vi "jl-script abs path.vi"(8 "error in (no error)":errorcluster, 10 "Base path (not a path)":path=path "", 11 "Julia user functions script":path) -> (0 "error out":errorcluster, 3 "script abs path":path)   [LabVIEW 2018, in "LV-0mq-Julia_roundtrip-lib.lvlib"]
doc: "If abs path is connected, this VI only checks if this file exists and puts the path through.\nFor a relative path, the abs path is constructed using the base path. \nIf base path not connected, the containing folder is assumed to be the \"jl-scripts\" folder in this LabVIEW library."
uses:
  LV-0mq-Julia_roundtrip-lib.lvlib
  <vilib>/Utility/error.llb/Error Cluster From Error Code.vi
  <vilib>/ErrorRing/Error Ring.xnode
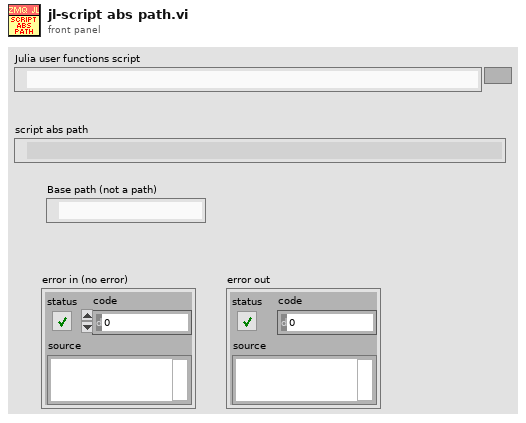
[diagram p1: front panel]
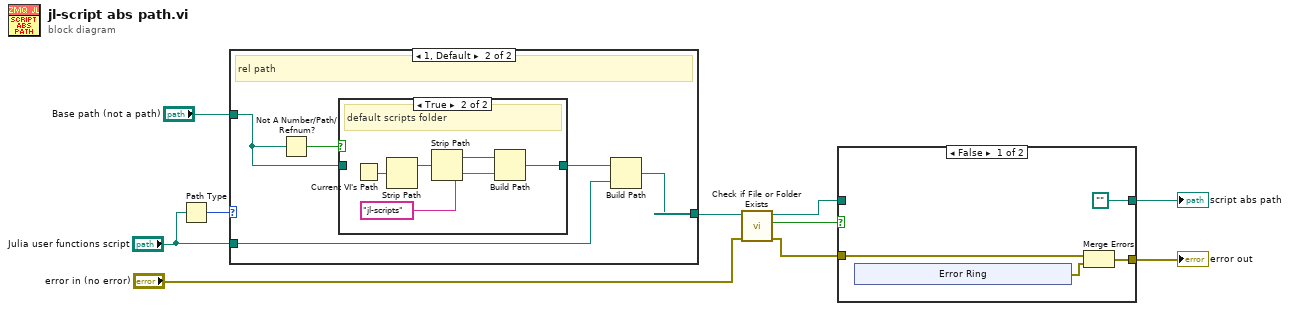
[diagram p0: block diagram]
diagram:
  n1 = Path Type(1:"Julia user functions script") -> (0:w3:i16)
  n2 = case shown="1, Default" w3 {
    tunnel: [w11 w16] -> w8
    tunnel: "Julia user functions script" -> [w11 w15]
    tunnel: "Base path (not a path)" -> [_ w12]
    frame 0 {
      # "abs path"
    }
    frame 1, Default {
      # "rel path"
      n3 = Not A Number/Path/Refnum?(number/path/refnum=w12) -> (NaN/Path/Refnum?=w14:bool)
      n4 = case shown="True" w14 {
        tunnel: [w17 w18] -> w13
        tunnel: w12 -> [w17 _]
        frame False {
          # "base path givem"
        }
        frame True {
          # "default scripts folder"
          n5 = Current VI's Path() -> (path=w22:path)
          n6 = Strip Path(path=w22) -> (stripped path=w21:path)  [unwired: 1 out]
          n7 = Strip Path(path=w21) -> (stripped path=w20:path)  [unwired: 1 out]
          n8 = Build Path(base path=w20, name or relative path="jl-scripts") -> (appended path=w18:path)
        }
      }
      n9 = Build Path(base path=w13, name or relative path=w15) -> (appended path=w16:path)
    }
  }
  n10 = call <vilib>:"Check if File or Folder Exists.vi"("error in (no error)"="error in (no error)", "path"=w8) -> ("error out"=w7:errorcluster, "file or folder exists?"=w10:bool, "dup path"=w9:path)  [unwired: 7 in]
  n11 = case shown="False" w10 {
    tunnel: w9 -> [_ w33]
    tunnel: [w25 w32] -> w4
    tunnel: w7 -> [w24 w32]
    tunnel: [path "" w33] -> w5
    frame False {
      n12 = xnode "Error Ring"() -> ("error out"=w26:errorcluster)
      n13 = Merge Errors(w24, w26) -> (w25:errorcluster)
    }
    frame True {
      # "script file exists"
    }
  }
  "script abs path" <- w5
  "error out" <- w4
